vi "cla.vi"() -> ()   [LabVIEW 2013]
uses:
  <vilib>/gmath/NI_Gmath.lvlib
panel:
  in  "Array":void[][][][](array[numeric])
  in  "fahrenheit 2":dbl(slide) scale=0.0..10.0
  in  "celsius":dbl(slide) scale=0.0..1.0
  in  "Digital Data":digitaldata
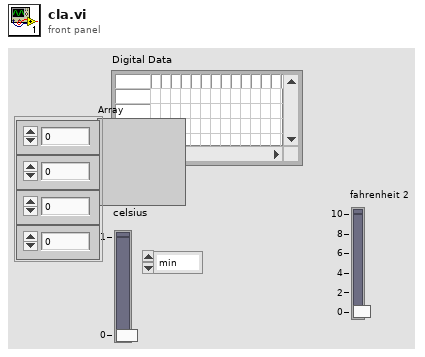
[diagram p1: front panel]
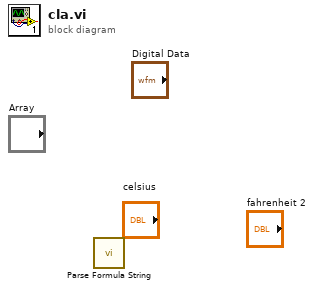
[diagram p0: block diagram]
diagram:
  n1 = call <vilib>:"Parse Formula String.vi"() -> ()  [unwired: 2 in, 2 out]
